vi "test_RS-xxx Read.vi"(8 "error in (no error)":errorcluster, 11 "TestCase in":refnum<class "Serial Protocols Tests.lvclass">) -> (0 "error out":errorcluster, 3 "TestCase out":refnum<class "Serial Protocols Tests.lvclass">)   [LabVIEW 2019, in "Serial Protocols Tests.lvclass"]
uses:
  Serial Protocols Tests.lvclass
  Listener/Listener.lvclass
  Listener/ListenerClassControls/Operation.ctl
  RS-xxx/RS-xxx.lvclass
  D:/GitRepository/niveristand-instrument-addon-classes/Source/Protocols/Protocol Parent/Protocol Parent.lvclass
  Protocol Parent/Methods/Read Parameter.ctl
  <vilib>/Platform/TimedLoop/XDataNode/timing_clust.ctl
  <vilib>/Platform/TimedLoop/XDataNode/nitl_modes.ctl
  <vilib>/Platform/TimedLoop/XDataNode/wakeup.ctl
  RS-xxx/RS-xxx.lvclass/RS-xxx.ctl
  <vilib>/platform/TimedLoop/XDataNode/XDataNode.xnode
  <vilib>/addons/_JKI Toolkits/VI Tester/TestCase.llb/TestCase.lvclass
  <vilib>/Platform/TimedLoop/XDataNode/XDNodeRunTimeDep.lvlib
  Protocol Parent/Protocol Parent.lvclass
  C:/Program Files (x86)/National Instruments/LabVIEW 2019/vi.lib/addons/_JKI Toolkits/VI Tester/TestCase.llb/TestCase.lvclass
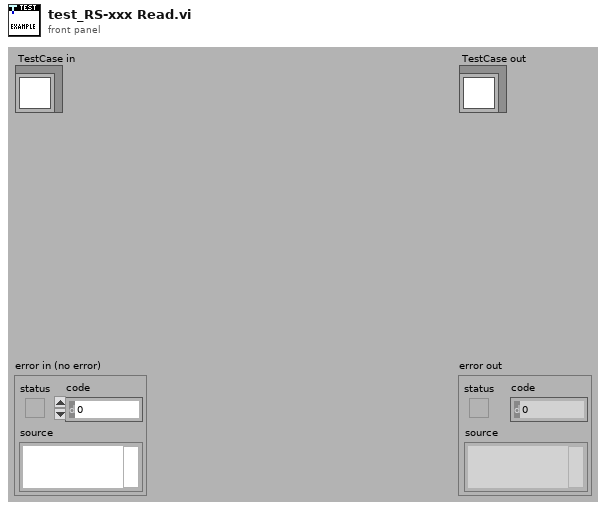
[diagram p1: front panel]
types:
  T1 = typedef "Protocols.lvlib/Protocol Parent.lvclass/Read Parameter.ctl" = cluster{"Wait Type":enum16{"Byte Count", "Wait sec"}, "Wait Value":dbl}
  T2 = typedef "Listener.lvclass/Operation.ctl" = enum16{"Read", "Write"}
  T3 = typedef "XDNodeRunTimeDep.lvlib/timing_clust.ctl" = cluster{"Expected End [f-1]":u64, "Actual End [f-1]":u64, "Finished Late? [f-1]":bool, "Expected End [i-1]":u64, "Actual End [i-1]":u64, "Finished Late? [i-1]":bool, "Expected Start [i]":u64, "Actual Start [i]":u64, "Expected Start [f]":u64, "Actual Start [f]":u64, "Source Name":string, "Structure Name":string, "Period":i64, "Deadline":i64, "Offset":i64, "Start":i64, "Priority":i32, "Timeout":i32, "Mode":T4, "Wakeup Reason":T5, "Error":errorcluster, "Source Type":string, "Secondary Source Type":string, "Global End Time":u64, "Global Start Time":u64, "Frame Duration":u64, "Iteration Duration":u64, "Assigned CPU":i32, "I/O Scan Engine Mode":u32}
  T4 = typedef "XDNodeRunTimeDep.lvlib/nitl_modes.ctl" = enum32{"No Change", "Process missed periods, maintain original phase", "Discard missed periods, maintain original phase", "Process missed periods, ignore original phase", "Discard missed periods, ignore original phase"}
  T5 = typedef "XDNodeRunTimeDep.lvlib/wakeup.ctl" = enum32{"Normal", "Aborted", "Asynchronous wakeup", "Timing source error", "Timed loop error", "Timeout"}
  T6 = typedef "Listener.lvclass/RS-xxx Data Structure.ctl" = cluster{"Protocol Port Ref":refnum<visa-resource-name>, "Listener Port Ref":refnum<visa-resource-name>, "Virtual COM Port Settings 1":cluster{"Port":string, "Baud Rate":u32, "Data Bits":u16, "Parity":enum16{"None", "Odd", "Even", "Mark", "Space"}, "Stop Bits":u16, "Flow Control":u16, "XON":enum16{"NUL", "SOH", "STX", "ETX", "EOT", "ENQ", "ACK", "BEL", "BS", "HT", "LF", "VT", "FF", "CR", "SO", "SI", "DLE", "DC1", "DC2", "DC3", "DC4", "NAK", "SYN", "ETB", "CAN", "EM", "SUB", "ESC", "FS", "GS", "RS", "US", "SP", "!", "\"", "#", "$", "%", "&", "'", "(", ")", "*", "+", ",", "- (-)", ".", "/", "0", "1", "2", "3", "4", "5", "6", "7", "8", "9", ":", ";", "<", "=", ">", "?", "@", "A", "B", "C", "D", "E", "F", "G", "H", "I", "J", "K", "L", "M", "N", "O", "P", "Q", "R", "S", "T", "U", "V", "W", "X", "Y", "Z", "[", "\\", "]", "^", "_", "`", "a", "b", "c", "d", "e", "f", "g", "h", "i", "j", "k", "l", "m", "n", "o", "p", "q", "r", "s", "t", "u", "v", "w", "x", "y", "z", "{", "|", "}", "~"}, "XOFF":enum16{"NUL", "SOH", "STX", "ETX", "EOT", "ENQ", "ACK", "BEL", "BS", "HT", "LF", "VT", "FF", "CR", "SO", "SI", "DLE", "DC1", "DC2", "DC3", "DC4", "NAK", "SYN", "ETB", "CAN", "EM", "SUB", "ESC", "FS", "GS", "RS", "US", "SP", "!", "\"", "#", "$", "%", "&", "'", "(", ")", "*", "+", ",", "- (-)", ".", "/", "0", "1", "2", "3", "4", "5", "6", "7", "8", "9", ":", ";", "<", "=", ">", "?", "@", "A", "B", "C", "D", "E", "F", "G", "H", "I", "J", "K", "L", "M", "N", "O", "P", "Q", "R", "S", "T", "U", "V", "W", "X", "Y", "Z", "[", "\\", "]", "^", "_", "`", "a", "b", "c", "d", "e", "f", "g", "h", "i", "j", "k", "l", "m", "n", "o", "p", "q", "r", "s", "t", "u", "v", "w", "x", "y", "z", "{", "|", "}", "~"}, "End Read on Termination Character":bool, "End Write on Termination Character":bool, "Termination Character":u8}, "Virtual COM Port Settings 2":cluster{"Port":string, "Baud Rate":u32, "Data Bits":u16, "Parity":enum16{"None", "Odd", "Even", "Mark", "Space"}, "Stop Bits":u16, "Flow Control":u16, "XON":enum16{"NUL", "SOH", "STX", "ETX", "EOT", "ENQ", "ACK", "BEL", "BS", "HT", "LF", "VT", "FF", "CR", "SO", "SI", "DLE", "DC1", "DC2", "DC3", "DC4", "NAK", "SYN", "ETB", "CAN", "EM", "SUB", "ESC", "FS", "GS", "RS", "US", "SP", "!", "\"", "#", "$", "%", "&", "'", "(", ")", "*", "+", ",", "- (-)", ".", "/", "0", "1", "2", "3", "4", "5", "6", "7", "8", "9", ":", ";", "<", "=", ">", "?", "@", "A", "B", "C", "D", "E", "F", "G", "H", "I", "J", "K", "L", "M", "N", "O", "P", "Q", "R", "S", "T", "U", "V", "W", "X", "Y", "Z", "[", "\\", "]", "^", "_", "`", "a", "b", "c", "d", "e", "f", "g", "h", "i", "j", "k", "l", "m", "n", "o", "p", "q", "r", "s", "t", "u", "v", "w", "x", "y", "z", "{", "|", "}", "~"}, "XOFF":enum16{"NUL", "SOH", "STX", "ETX", "EOT", "ENQ", "ACK", "BEL", "BS", "HT", "LF", "VT", "FF", "CR", "SO", "SI", "DLE", "DC1", "DC2", "DC3", "DC4", "NAK", "SYN", "ETB", "CAN", "EM", "SUB", "ESC", "FS", "GS", "RS", "US", "SP", "!", "\"", "#", "$", "%", "&", "'", "(", ")", "*", "+", ",", "- (-)", ".", "/", "0", "1", "2", "3", "4", "5", "6", "7", "8", "9", ":", ";", "<", "=", ">", "?", "@", "A", "B", "C", "D", "E", "F", "G", "H", "I", "J", "K", "L", "M", "N", "O", "P", "Q", "R", "S", "T", "U", "V", "W", "X", "Y", "Z", "[", "\\", "]", "^", "_", "`", "a", "b", "c", "d", "e", "f", "g", "h", "i", "j", "k", "l", "m", "n", "o", "p", "q", "r", "s", "t", "u", "v", "w", "x", "y", "z", "{", "|", "}", "~"}, "End Read on Termination Character":bool, "End Write on Termination Character":bool, "Termination Character":u8}, "Data":string, "Data Length":u32}
  T7 = cluster{"Port":string, "Baud Rate":u32, "Data Bits":u16, "Parity":enum16{"None", "Odd", "Even", "Mark", "Space"}, "Stop Bits":u16, "Flow Control":u16, "XON":enum16{"NUL", "SOH", "STX", "ETX", "EOT", "ENQ", "ACK", "BEL", "BS", "HT", "LF", "VT", "FF", "CR", "SO", "SI", "DLE", "DC1", "DC2", "DC3", "DC4", "NAK", "SYN", "ETB", "CAN", "EM", "SUB", "ESC", "FS", "GS", "RS", "US", "SP", "!", "\"", "#", "$", "%", "&", "'", "(", ")", "*", "+", ",", "- (-)", ".", "/", "0", "1", "2", "3", "4", "5", "6", "7", "8", "9", ":", ";", "<", "=", ">", "?", "@", "A", "B", "C", "D", "E", "F", "G", "H", "I", "J", "K", "L", "M", "N", "O", "P", "Q", "R", "S", "T", "U", "V", "W", "X", "Y", "Z", "[", "\\", "]", "^", "_", "`", "a", "b", "c", "d", "e", "f", "g", "h", "i", "j", "k", "l", "m", "n", "o", "p", "q", "r", "s", "t", "u", "v", "w", "x", "y", "z", "{", "|", "}", "~"}, "XOFF":enum16{"NUL", "SOH", "STX", "ETX", "EOT", "ENQ", "ACK", "BEL", "BS", "HT", "LF", "VT", "FF", "CR", "SO", "SI", "DLE", "DC1", "DC2", "DC3", "DC4", "NAK", "SYN", "ETB", "CAN", "EM", "SUB", "ESC", "FS", "GS", "RS", "US", "SP", "!", "\"", "#", "$", "%", "&", "'", "(", ")", "*", "+", ",", "- (-)", ".", "/", "0", "1", "2", "3", "4", "5", "6", "7", "8", "9", ":", ";", "<", "=", ">", "?", "@", "A", "B", "C", "D", "E", "F", "G", "H", "I", "J", "K", "L", "M", "N", "O", "P", "Q", "R", "S", "T", "U", "V", "W", "X", "Y", "Z", "[", "\\", "]", "^", "_", "`", "a", "b", "c", "d", "e", "f", "g", "h", "i", "j", "k", "l", "m", "n", "o", "p", "q", "r", "s", "t", "u", "v", "w", "x", "y", "z", "{", "|", "}", "~"}, "End Read on Termination Character":bool, "End Write on Termination Character":bool, "Termination Character":u8}
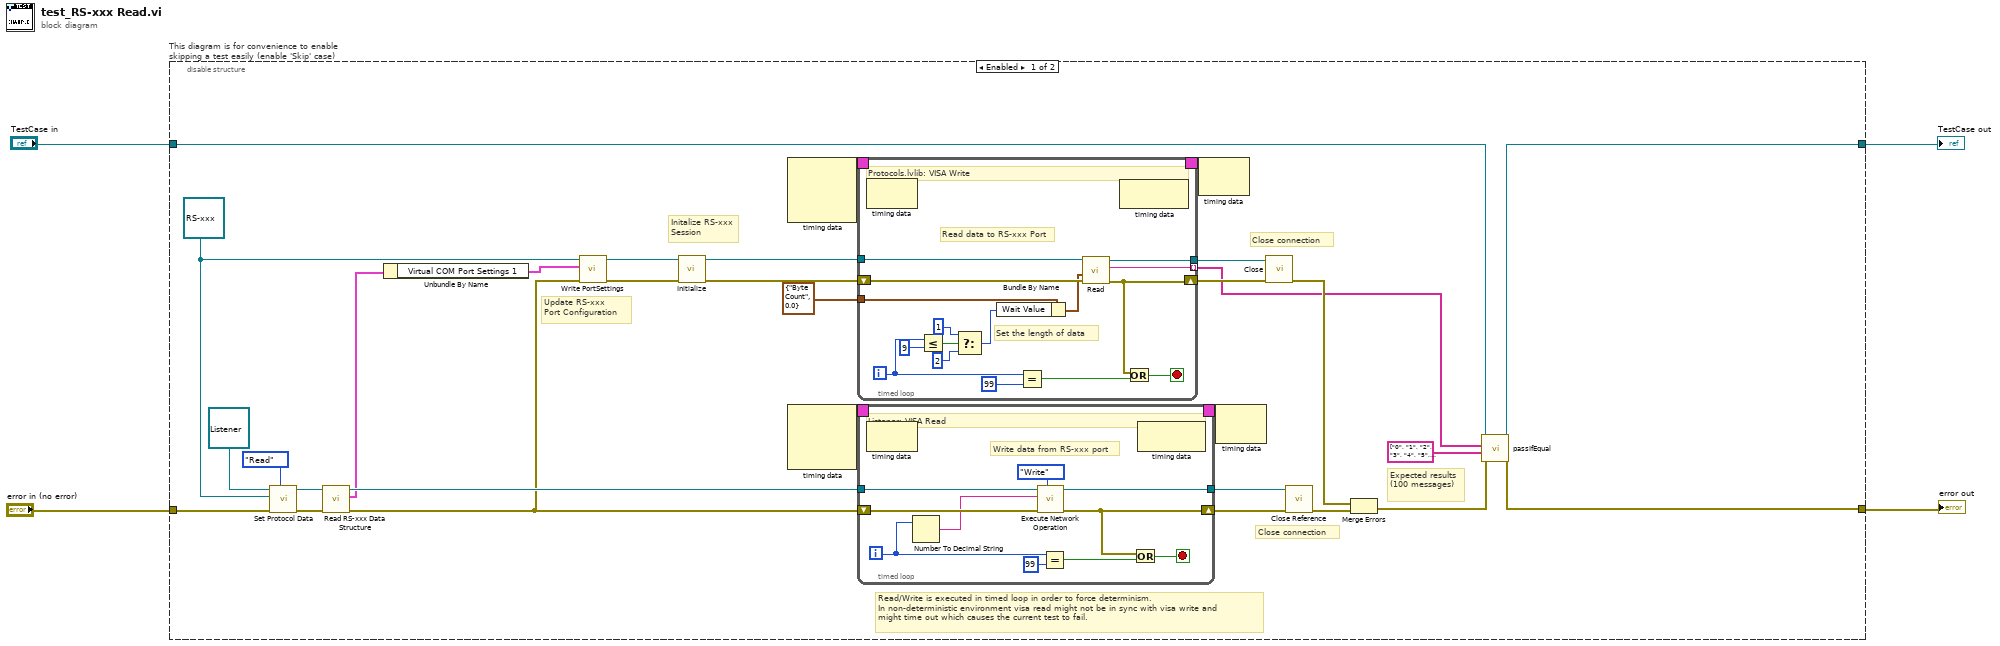
[diagram p0: block diagram]
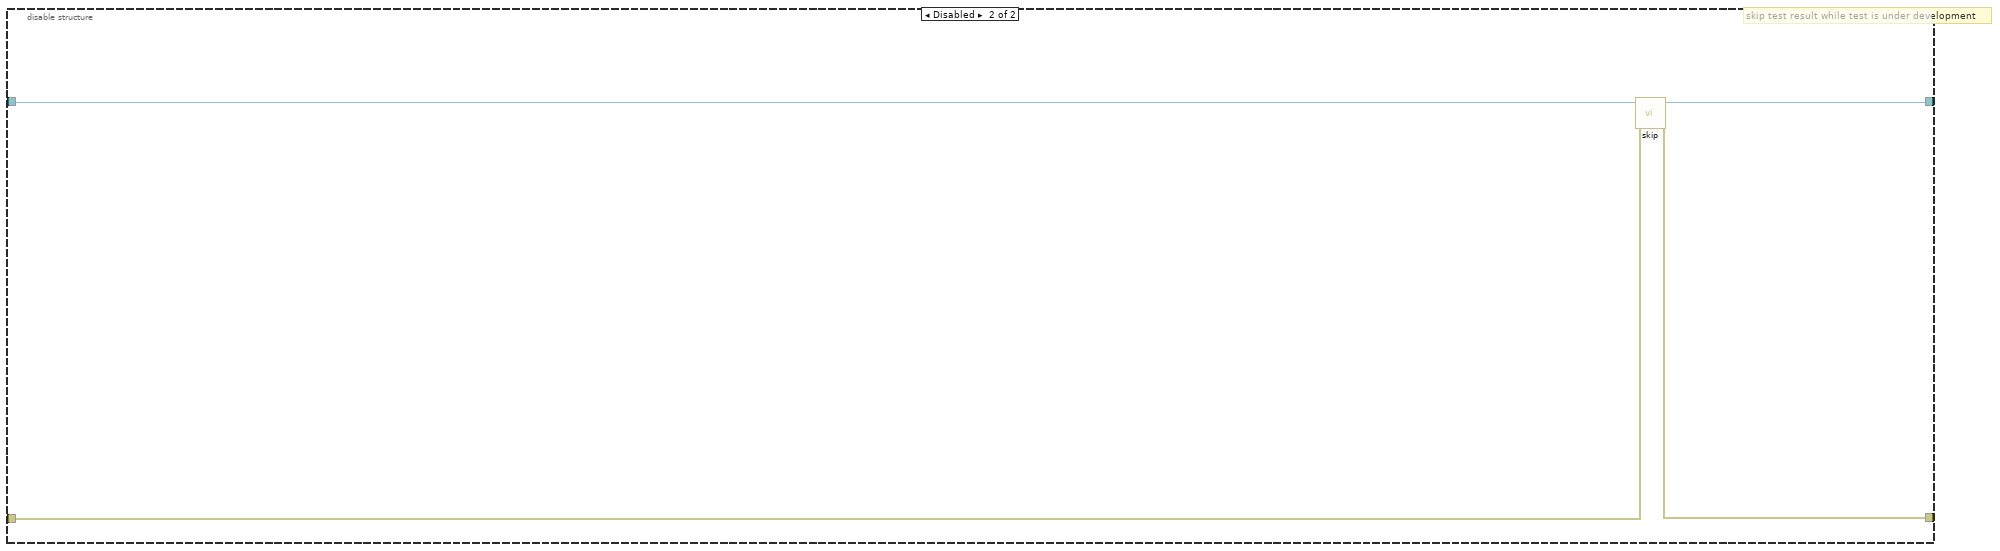
[diagram p2: hidden frame]
diagram:
  n1 = disable-structure "This diagram is for convenience to enable skipping a test easily (enable 'Skip' case)" shown="Enabled" {
    disable-tunnel: "TestCase in" -> [w35 w73]
    disable-tunnel: [w34 w71] -> w1
    disable-tunnel: [w33 w72] -> w3
    disable-tunnel: "error in (no error)" -> [w29 w70]
    frame Enabled {
      w16 = refnum<class "RS-xxx.lvclass"> refnum ("Protocols.lvlib:RS-xxx.lvclass")
      # "Update RS-xxx \nPort Configuration"
      # "Initalize RS-xxx\nSession"
      # "Close connection"
      # "Close connection"
      # "Read/Write is executed in timed loop in order to force determinism.\nIn non-deterministic environment visa read might not be in sync with visa write and\nmight time out which causes the current test to fail."
      # "Expected results\n(100 messages)"
      n2 = call "Set Protocol Data.vi"("Operation"=Operation."Read", "error in (no error)"=w29, "Protocols.lvlib:Protocol Parent.lvclass"=w16, "Listener In.lvclass"=refnum<class "Listener.lvclass"> refnum ("Listener.lvclass")) -> ("error out"=w18:errorcluster, "Listener Out.lvclass"=w19:refnum<class "Listener.lvclass">)  [unwired: 6 in]
      n3 = call-dynamic "Read RS-xxx Data Structure.vi"("error in (no error)"=w18, "Listener in"=w19) -> ("error out"=w11:errorcluster, "RS-xxx Data Structure"=w10:T6, "Listener out"=w12:refnum<class "Listener.lvclass">)  [unwired: 7 in]
      n4 = Unbundle By Name(w10) -> ("Virtual COM Port Settings 1"=w9:T7)
      n5 = call "Write PortSettings.vi"("error in (no error)"=w11, "Cluster"=w9, "RS232 in"=w16) -> ("error out"=w17:errorcluster, "RS232 out"=w15:refnum<class "RS-xxx.lvclass">)  [unwired: 7 in]
      n6 = call-dynamic "Initialize.vi"("error in (no error)"=w17, "RS232 in"=w15) -> ("error out"=w14:errorcluster, "RS232 out"=w13:refnum<class "RS-xxx.lvclass">)  [unwired: 8 in]
      n7 = node-c288() -> (w23:T3)  [unwired: 3 in]
      n8 = node-c288() -> (w21:T3)  [unwired: 3 in]
      n9 = timed-loop {
        shift-right: [w50] -> w26
        shift-left: w14 -> [w62]
        timing: w23 -> [_]
        timing-out: [_] -> w22
        tunnel: w13 -> [w61]
        tunnel: T1 {"Wait Type"=enum."Byte Count", "Wait Value"=0.0} ("Read Parameter") -> [w55]
        tunnel: [w52] -> w7
        tunnel: [w51] -> w5 mode=indexing
        i -> [w56]
        stop <- w63 stop-if-true
        # "Set the length of data"
        # "Read data to RS-xxx Port"
        # "Protocols.lvlib: VISA Write"
        n10 = node-c288() -> ()  [unwired: 1 in, 1 out]
        n11 = Less Or Equal?(x=w56, y=9) -> (x <= y?=w59:bool)
        n12 = Select(t=u32 1, s=w59, f=u32 2) -> (s? t:f=w54:u32)
        n13 = Bundle By Name(cluster=w55, "Wait Value"=w54) -> (w53:T1)
        n14 = Equal?(x=w56, y=99) -> (x = y?=w65:bool)
        n15 = call-dynamic "Read.vi"("error in (no error)"=w62, "Variant"=w53, "RS232 in"=w61) -> ("error out"=w50:errorcluster, "String"=w51:string, "RS232 out"=w52:refnum<class "RS-xxx.lvclass">)  [unwired: 6 in]
        n16 = node-c288() -> ()  [unwired: 1 in, 1 out]
        n17 = Or(x=w50, y=w65) -> (x .or. y?=w63:bool)
      }
      n18 = timed-loop {
        shift-right: [w41] -> w24
        shift-left: w11 -> [w38]
        tunnel: [w40] -> w25
        timing: w21 -> [_]
        timing-out: [_] -> w20
        tunnel: w12 -> [w39]
        i -> [w37]
        stop <- w42 stop-if-true
        # "Write data from RS-xxx port"
        # "Listener: VISA Read"
        n19 = node-c288() -> ()  [unwired: 1 in, 1 out]
        n20 = Number To Decimal String(number=w37) -> (decimal integer string=w36:string)  [unwired: 1 in]
        n21 = call "Execute Network Operation.vi"("Operation"=Operation."Write", "error in (no error)"=w38, "Message"=w36, "Listener In.lvclass"=w39) -> ("error out"=w41:errorcluster, "Listener Out.lvclass"=w40:refnum<class "Listener.lvclass">)  [unwired: 6 in]
        n22 = Equal?(x=w37, y=99) -> (x = y?=w43:bool)
        n23 = Or(x=w41, y=w43) -> (x .or. y?=w42:bool)
        n24 = node-c288() -> ()  [unwired: 1 in, 1 out]
      }
      n25 = node-c288(w22) -> ()  [unwired: 1 out]
      n26 = node-c288(w20) -> ()  [unwired: 1 out]
      n27 = call-dynamic "Close.vi"("error in (no error)"=w26, "RS232 in"=w7) -> ("error out"=w28:errorcluster)  [unwired: 8 in, 1 out]
      n28 = call "Close Reference.vi"("error in (no error)"=w24, "Listener In.lvclass"=w25) -> ("error out"=w27:errorcluster)  [unwired: 9 in]
      n29 = Merge Errors(w28, w27) -> (w30:errorcluster)
      n30 = call-dynamic "passIfEqual.vi"("error in (no error)"=w30, "y"=string[] ["0", "1", "2", "3", "4", "5", "6", "7", "8", "9", "10", "11", "12", "13", "14", "15", "16", "17", "18", "19", "20", "21", "22", "23", "24", "25", "26", "27", "28", "29", "30", "31", "32", "33", "34", "35", "36", "37", "38", "39", "40", "41", "42", "43", "44", "45", "46", "47", "48", "49", "50", "51", "52", "53", "54", "55", "56", "57", "58", "59", "60", "61", "62", "63", "64", "65", "66", "67", "68", "69", "70", "71", "72", "73", "74", "75", "76", "77", "78", "79", "80", "81", "82", "83", "84", "85", "86", "87", "88", "89", "90", "91", "92", "93", "94", "95", "96", "97", "98", "99"] ("Array"), "x"=w5, "TestCase in"=w35) -> ("error out"=w33:errorcluster, "TestCase out"=w34:refnum<class "Serial Protocols Tests.lvclass">)  [unwired: 6 in]
    }
    frame Disabled {
      # "skip test result while test is under development"
      n31 = call <vilib>:"skip.vi"("error in (no error)"=w70, "TestCase in"=w73) -> ("error out"=w72:errorcluster, "TestCase out"=w71:refnum<class "Serial Protocols Tests.lvclass">)  [unwired: 8 in]
    }
  }
  "error out" <- w3
  "TestCase out" <- w1
